vi "Quaternion_GetLAll.vi"(11 "Quaternion":T1={"R"=1.0, "V"=[0.0, 0.0, 0.0]}) -> (0 "Z":dbl, 1 "Y":dbl, 2 "X":dbl, 3 "W":dbl=1.0)   [LabVIEW 2019, in "Trajectory_Library.lvlib"]
doc: "Convenience constructors that takes in x and y values directly instead of having to construct a Translation2d.\n\nParameters:\n - X- The x component of the translational component of the pose.\n - Y - The y component of the translational component of the pose.\n - Rotation (Heading) - The rotational component of the pose.\n\nReturns:\n - OUT POSE - Output POSE"
uses:
  QUATERNION.ctl
  Trajectory_Library.lvlib
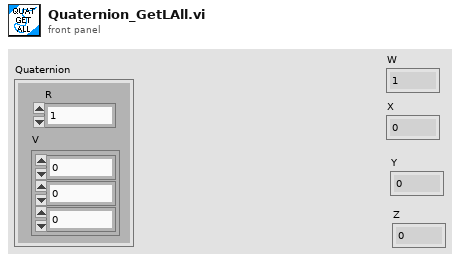
[diagram p1: front panel]
types:
  T1 = typedef "Trajectory_Library.lvlib/QUATERNION.ctl" = cluster{"R":dbl, "V":dbl[]}
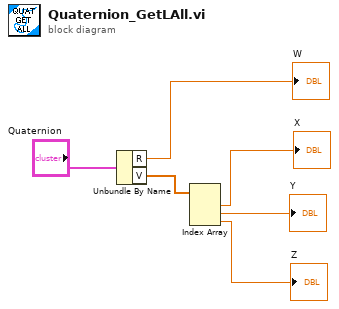
[diagram p0: block diagram]
diagram:
  n1 = Unbundle By Name("Quaternion") -> ("R"=→"W":dbl, "V"=w4:dbl[])
  n2 = Index Array(array=w4) -> (element #1=→"X":dbl, element #2=→"Y":dbl, element #3=→"Z":dbl)  [unwired: 3 in]
